vi "WriteBufferError (RelativeCode).vi"(8 "error in (no error)":errorcluster, 10 "Error message":string, 11 "Relative error code (548600 + input)":i32) -> (0 "error out":errorcluster)   [LabVIEW 2013, in "CircularBuffer.lvlib" / "VariantBuffer.lvclass"]
uses:
  VariantBuffer.lvclass
  buffer-errors -- ring.ctl
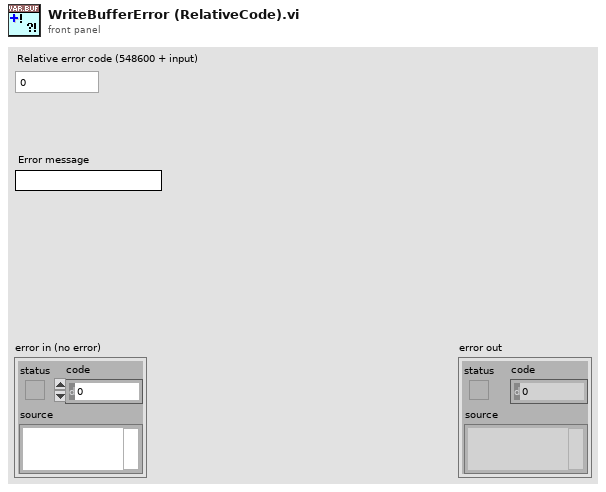
[diagram p1: front panel]
types:
  T1 = typedef "CircularBuffer.lvlib/VariantBuffer.lvclass/buffer-errors -- ring.ctl" = i32
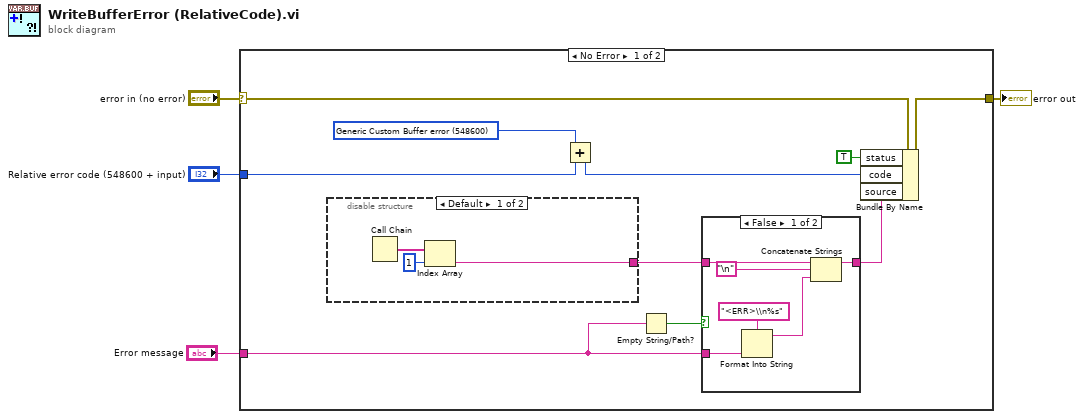
[diagram p0: block diagram]
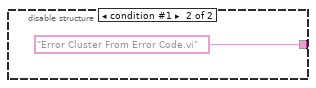
[diagram p3: hidden frame]
diagram:
  n1 = case shown="No Error" "error in (no error)" {
    selector: "error in (no error)" -> [w12 w26]
    tunnel: [w14 w26] -> w4
    tunnel: "Relative error code (548600 + input)" -> [w13 _]
    tunnel: "Error message" -> [w7 _]
    frame No Error {
      w10 = T1 548600 items=["No error"=0, "Generic Buffer error"=548500, "Generic Custom Buffer error"=548600, "Buffer is full"=548501, "Buffer is empty"=548502, "Buffer size cannot be 0"=548503, "Buffer reference is invalid"=548504, "Buffer event reference invalid"=548505, "Buffer Type not supported"=548506, "Not enough space in the buffer for this operation"=548507] ("buffer-errors")
      n2 = disable-structure shown="Default" {
        disable-tunnel: [w22 "Error Cluster From Error Code.vi" ("source")] -> w6
        frame condition #0 (active) {
          n3 = Call Chain() -> (call chain=w23:string[])
          n4 = Index Array(array=w23, index=1) -> (element=w22:string)
        }
        frame condition #1 {
        }
      }
      n5 = Add(x=w10, y=w13) -> (x+y=w9:T1)
      n6 = Empty String/Path?(string/path=w7) -> (empty?=w8:bool)
      n7 = case shown="False" w8 {
        tunnel: w7 -> [w16 _]
        tunnel: [w19 w21] -> w5
        tunnel: w6 -> [w20 w21]
        frame False {
          n8 = Format Into String(format string="<ERR>\\n%s", w16) -> (resulting string=w15:string)  [unwired: 2 in, 1 out]
          n9 = Concatenate Strings(w20, "\n", w15) -> (w19:string)
        }
        frame True {
        }
      }
      n10 = Bundle By Name(cluster=w12, "status"=TRUE, "code"=w9, "source"=w5) -> (w14:errorcluster)
    }
    frame Error {
      # "Upstream Error. Do not replace"
    }
  }
  "error out" <- w4
